vi "Abort LowMaster.vi"   [LabVIEW 2021]
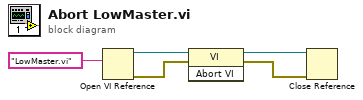
[diagram p0: block diagram]
diagram:
  n1 = Open VI Reference(vi path="LowMaster.vi") -> (vi reference=w4:refnum<vi>, error out=w1:errorcluster)  [unwired: 5 in]
  n2 = invoke class="VI" method="Abort VI"(reference=w4, error in=w1) -> (reference out=w3:refnum<vi>, error out=w2:errorcluster)  [unwired: 1 in, 1 out]
  n3 = Close Reference(reference=w3, error in (no error)=w2) -> ()  [unwired: 1 out]
